vi "programa5.vi"() -> ()   [LabVIEW 2011]
panel:
  out "Personas":dbl
  in  "Planta":u16(ring) items=["Planta #1", "Planta #2", "Planta #3"]
  out "A/c":bool
  out "Temperatura":i32(slide) scale=0.0..60.0
  # "Se genera la temperatura entre 1-60,\nse selecciona la planta usando el menu ring,\nluego se genera el numero de personas entre 1-50"
  # "planta 1 si hay mas de 25 personas y la temperatura\nes mayor a 22 se enciende el A/C\n\nplanta 2 si hay mas de 30 personas y la temperatura\nes mayor a 27 se enciende el A/C\n\nplanta 3 si hay mas de 20 personas y la temperatura\nes mayor a 29 se enciende el A/C"
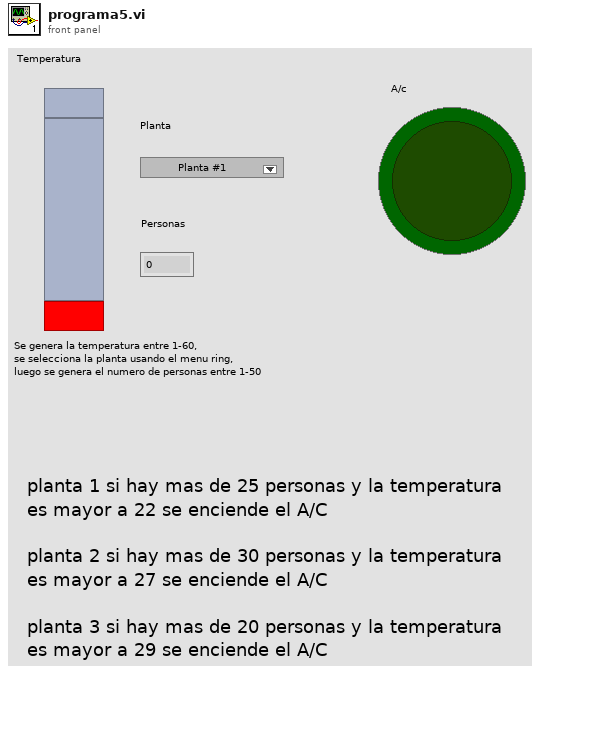
[diagram p1: front panel]
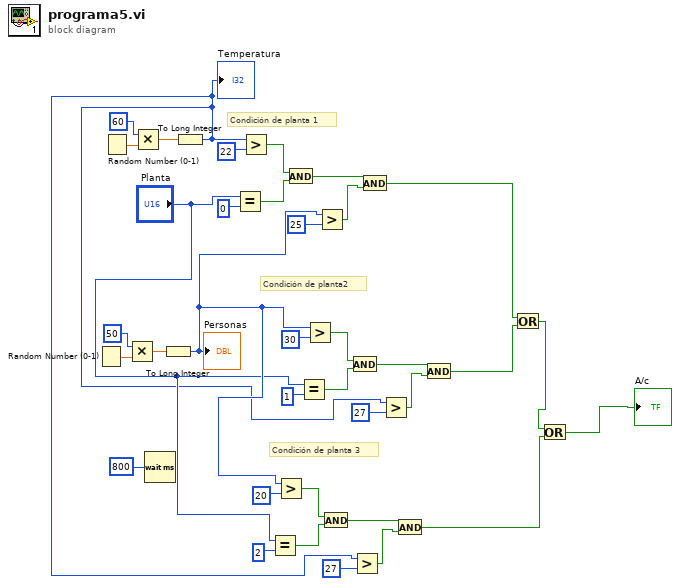
[diagram p0: block diagram]
diagram:
  # "Condición de planta 3"
  # "Condición de planta 1"
  # "Condición de planta2"
  n1 = Random Number (0-1)() -> (number: 0 to 1=w32:dbl)
  n2 = Random Number (0-1)() -> (number: 0 to 1=w35:dbl)
  n3 = Multiply(x=50, y=w32) -> (x*y=w33:dbl)
  n4 = Multiply(x=60, y=w35) -> (x*y=w34:dbl)
  n5 = Wait (ms)(milliseconds to wait=u32 800) -> ()  [unwired: 1 out]
  n6 = To Long Integer(number=w33) -> (32bit integer=w8:i32)
  "Personas" <- w8
  n7 = To Long Integer(number=w34) -> (32bit integer=w6:i32)
  "Temperatura" <- w6
  n8 = Equal?(x="Planta", y=u16 0) -> (x = y?=w25:bool)
  n9 = Greater?(x=w6, y=22) -> (0:w26:bool)
  n10 = Equal?(x="Planta", y=u16 2) -> (x = y?=w11:bool)
  n11 = Greater?(x=w8, y=20) -> (0:w12:bool)
  n12 = And(x=w26, y=w25) -> (x .and. y?=w24:bool)
  n13 = Equal?(x="Planta", y=u16 1) -> (x = y?=w20:bool)
  n14 = Greater?(x=w8, y=30) -> (0:w19:bool)
  n15 = Greater?(x=w8, y=25) -> (0:w23:bool)
  n16 = And(x=w12, y=w11) -> (x .and. y?=w10:bool)
  n17 = And(x=w19, y=w20) -> (x .and. y?=w21:bool)
  n18 = Greater?(x=w6, y=27) -> (0:w9:bool)
  n19 = And(x=w24, y=w23) -> (x .and. y?=w5:bool)
  n20 = Greater?(x=w6, y=27) -> (0:w22:bool)
  n21 = And(x=w10, y=w9) -> (x .and. y?=w3:bool)
  n22 = And(x=w21, y=w22) -> (x .and. y?=w4:bool)
  n23 = Or(x=w5, y=w4) -> (x .or. y?=w2:bool)
  n24 = Or(x=w2, y=w3) -> (x .or. y?=→"A/c":bool)
